vi "JSR SetPulse.vi"(8 "error in (no error)":errorcluster, 10 "JSR Pulse Settings":T1={"Damping"=52, "Pulse Energy Level"=1, "Pulser Impedance"=0, "Pulser Voltage (V)"=100} {"Pulser Voltage (V)" items=["100"=100, "125"=125, "150"=150, "175"=175, "200"=200, "225"=225, "250"=250, "275"=275, "300"=300, "325"=325, "350"=350, "375"=375, "400"=400, "425"=425, "450"=450, "475"=475]; "Pulser Impedance" items=["High z", "Low z"]; "Pulse Energy Level" items=["0 (Minimum)", "1", "2", "3 (Maximum)"]; "Damping" items=["331 Ohms"=331, "198 Ohms"=198, "142 Ohms"=142, "110 Ohms"=110, "92 Ohms"=92, "77 Ohms"=77, "67 Ohms"=67, "59 Ohms"=59, "52 Ohms"=52, "47 Ohms"=47, "43 Ohms"=43, "39 Ohms"=39, "37 Ohms"=37, "34 Ohms"=34, "32 Ohms"=32, "30 Ohms"=30]}, 11 "VISA Refnum in":refnum<visa-resource-name>) -> (0 "error out":errorcluster, 3 "VISA Refnum out":refnum<visa-resource-name>)   [LabVIEW 2022 SP3]
uses:
  Controls/JSR Pulse.ctl
  Controls/Damping.ctl
  Controls/Energy.ctl
  Controls/Z.ctl
  Controls/Volt.ctl
  PulserGlobals.vi
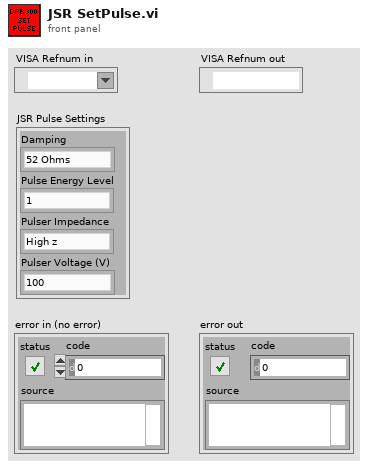
[diagram p1: front panel]
types:
  T1 = typedef "JSR Pulse.ctl" = cluster{"Damping":T2, "Pulse Energy Level":T3, "Pulser Impedance":T4, "Pulser Voltage (V)":T5}
  T2 = typedef "Damping.ctl" = i16
  T3 = typedef "Energy.ctl" = u16
  T4 = typedef "Z.ctl" = u16
  T5 = typedef "Volt.ctl" = i16
  T6 = cluster{"Energy (microJ)":u8, "Damping (In Ohm)":u8, "HP Filt(KHz) ":u16, "LP Filt (MHz)":u8, "Gain (db)":u8, "Atten (dB)":sgl}
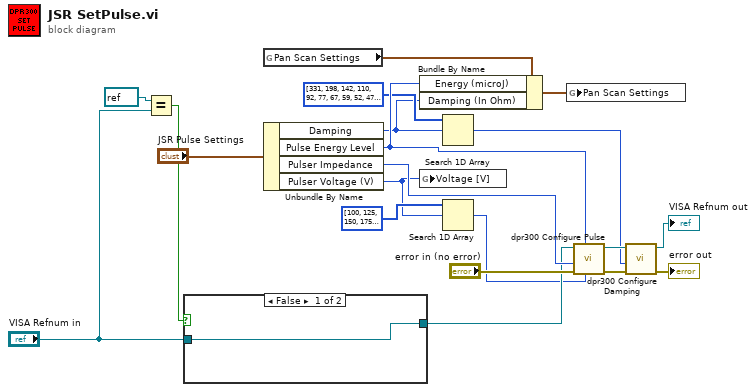
[diagram p0: block diagram]
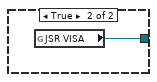
[diagram p2: hidden frame]
diagram:
  w5 = T2[] [331, 198, 142, 110, 92, 77, 67, 59, 52, 47, 43, 39, 37, 34, 32, 30] items=["331 Ohms"=331, "198 Ohms"=198, "142 Ohms"=142, "110 Ohms"=110, "92 Ohms"=92, "77 Ohms"=77, "67 Ohms"=67, "59 Ohms"=59, "52 Ohms"=52, "47 Ohms"=47, "43 Ohms"=43, "39 Ohms"=39, "37 Ohms"=37, "34 Ohms"=34, "32 Ohms"=32, "30 Ohms"=30]
  w6 = T5[] [100, 125, 150, 175, 200, 225, 250, 275, 300, 325, 350, 375, 400, 425, 450, 475] items=["100"=100, "125"=125, "150"=150, "175"=175, "200"=200, "225"=225, "250"=250, "275"=275, "300"=300, "325"=325, "350"=350, "375"=375, "400"=400, "425"=425, "450"=450, "475"=475]
  n1 = Equal?(x=refnum<visa-resource-name> refnum, y="VISA Refnum in") -> (x = y?=w12:bool)
  n2 = case shown="False" w12 {
    tunnel: [w21 w22] -> w11
    tunnel: "VISA Refnum in" -> [w21 _]
    frame False {
    }
    frame True {
      n3 = global read "PulserGlobals.vi" "JSR VISA"() -> (w22:refnum<visa-resource-name>)
    }
  }
  n4 = global read "PulserGlobals.vi" "Pan Scan Settings"() -> (w9:T6)
  n5 = Unbundle By Name("JSR Pulse Settings") -> ("Damping"=w1:T2, "Pulse Energy Level"=w7:T3, "Pulser Impedance"=w16:T4, "Pulser Voltage (V)"=w4:T5)
  n6 = Bundle By Name(cluster=w9, "Energy (microJ)"=w7, "Damping (In Ohm)"=w1) -> (w8:T6)
  n7 = global write "PulserGlobals.vi" "Voltage [V]"(w4) -> ()
  n8 = Search 1D Array(1D array=w5, element=w1) -> (index of element=w2:i32)  [unwired: 1 in]
  n9 = Search 1D Array(1D array=w6, element=w4) -> (index of element=w3:i32)  [unwired: 1 in]
  n10 = global write "PulserGlobals.vi" "Pan Scan Settings"(w8) -> ()
  n11 = call <instrlib>:"dpr300 Configure Pulse.vi"("Pulser Voltage (0: 100 V)"=w3, "Pulse Energy Level (2)"=w7, "error in (no error)"="error in (no error)", "Pulser Impedance (0: High z)"=w16, "VISA resource name"=w11) -> ("error out"=w17:errorcluster, "VISA resource name out"=w19:refnum<visa-resource-name>)  [unwired: 5 in]
  n12 = call <instrlib>:"dpr300 Configure Damping.vi"("error in (no error)"=w17, "Damping (8: 52 Ohms)"=w2, "VISA resource name"=w19) -> ("error out"=→"error out":errorcluster, "VISA resource name out"=→"VISA Refnum out":refnum<visa-resource-name>)  [unwired: 7 in]
